vi "Write Data.vi"(7 "TX.Data":T1 caption="Transmission Data" format="%.0x", 8 "error in (no error)":errorcluster, 11 "Low Speed in":refnum<class "Low Speed.lvclass">) -> (0 "error out":errorcluster, 3 "Low Speed out":refnum<class "Low Speed.lvclass">)   [LabVIEW 2020, in "Low Speed.lvclass"]
uses:
  Low Speed.lvclass
  C:/Users/kaiser.asan/OneDrive - SolitonTechnologies/LabVIEW/29.SDLC - I2C Driver/I2C Module/I2C Controller Module/Class/Transmission Mode/Parent/TX Speed.lvclass
  TypeDef/Transmission Data.ctl
  Low Speed.lvclass/Low Speed.ctl
  Parent/TX Speed.lvclass
  I2C Controller Lib.lvlib
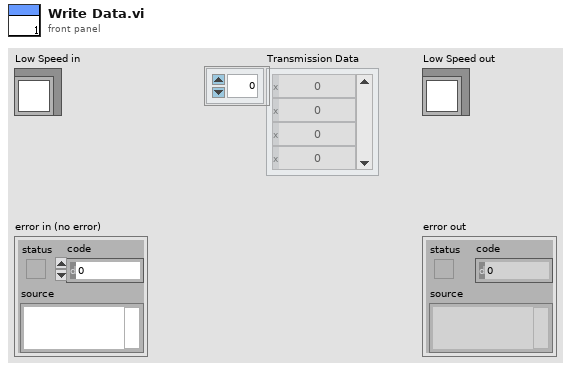
[diagram p1: front panel]
types:
  T1 = typedef "I2C Controller Lib.lvlib/Transmission Data.ctl" = u8[]
  T2 = typedef "I2C Controller Lib.lvlib/Timing Parameters Cluster.ctl" = cluster{"f_SCL(KHz)":u32, "t_HIGH (ns)":u32, "t_LOW (ns)":u32, "t_SU;STA (ns)":u32, "t_HD;STA (ns)":u32, "t_SU;DAT (ns)":u32, "t_HD;DAT (ns)":u32, "t_SU;STO (ns)":u32, "t_BUF (ns)":u32}
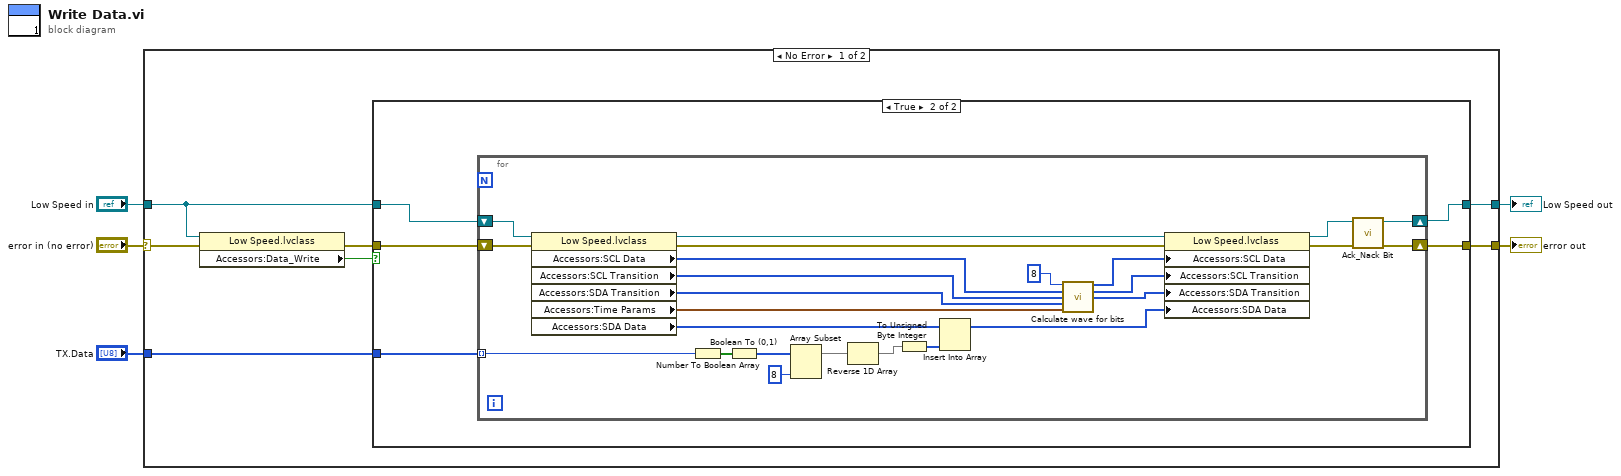
[diagram p0: block diagram]
diagram:
  n1 = case shown="No Error" "error in (no error)" {
    selector: "error in (no error)" -> [w12 w46]
    tunnel: [w11 w46] -> w5
    tunnel: [w9 w45] -> w3
    tunnel: "Low Speed in" -> [w8 w45]
    tunnel: "TX.Data" -> [w6 _]
    frame No Error {
      n2 = property class="Low Speed.lvclass"(reference=w8, error in=w12) -> (error out=w10:errorcluster, "Accessors:Data_Write"=w7:bool)  [unwired: 1 out]
      n3 = case shown="True" w7 {
        tunnel: [w13 w15] -> w11
        tunnel: w10 -> [w13 w19]
        tunnel: [w14 w16] -> w9
        tunnel: w8 -> [w14 w18]
        tunnel: w6 -> [_ w17]
        frame False {
        }
        frame True {
          n4 = for {
            tunnel: w17 -> [w31] mode=indexing
            shift-right: [w27] -> w15
            shift-left: w19 -> [w44]
            shift-right: [w28] -> w16
            shift-left: w18 -> [w41]
            n5 = property class="Low Speed.lvclass"(reference=w41, error in=w44) -> (reference out=w42:refnum<class "Low Speed.lvclass">, error out=w43:errorcluster, "Accessors:SCL Data"=w40:u8[], "Accessors:SCL Transition"=w39:u32[], "Accessors:SDA Transition"=w38:u32[], "Accessors:Time Params"=w37:T2, "Accessors:SDA Data"=w33:u8[])
            n6 = Number To Boolean Array(number=w31) -> (Boolean array=w25:bool[])
            n7 = Boolean To (0,1)(Boolean=w25) -> (0, 1=w24:i16[])
            n8 = Array Subset(array=w24, length=8) -> (w23:i16[])  [unwired: 1 in]
            n9 = Reverse 1D Array(array=w23) -> (reversed array=w21:i16[])
            n10 = To Unsigned Byte Integer(number=w21) -> (unsigned 8bit integer=w20:u8[])
            n11 = Insert Into Array(array=w33, new element=w20) -> (w32:u8[])  [unwired: 1 in]
            n12 = call "Calculate wave for bits.vi"("No. Of Bits"=8 ("x"), "SCL DATA IN"=w40, "SCL Transitions In"=w39, "SDA Transitions In"=w38, "Time Params"=w37) -> ("SCL DATA OUT"=w36:u8[], "SCL Transitions Out"=w35:u32[], "SDA Transitions Out"=w34:u32[])  [unwired: 8 in]
            n13 = property class="Low Speed.lvclass"(reference=w42, error in=w43, "Accessors:SCL Data"=w36, "Accessors:SCL Transition"=w35, "Accessors:SDA Transition"=w34, "Accessors:SDA Data"=w32) -> (reference out=w29:refnum<class "Low Speed.lvclass">, error out=w30:errorcluster)
            n14 = call-dynamic "Ack_Nack Bit.vi"("error in (no error)"=w30, "Low Speed in"=w29) -> ("error out"=w27:errorcluster, "Low Speed out"=w28:refnum<class "Low Speed.lvclass">)  [unwired: 8 in]
          }
        }
      }
    }
    frame Error {
    }
  }
  "error out" <- w5
  "Low Speed out" <- w3
